vi "LEBITplc.IGSetValue.vi"(0 "i ref in":refnum<vi>, 1 "Nickname in":string, 2 "index in":i32, 3 "value":dbl, 5 "error in (no error)":errorcluster) -> (13 "In Range?":bool, 14 "i ref out":refnum<vi>, 15 "Nicknames out":string[](array[string]), 16 "Index out":i32[](array[numeric]), 17 "values":dbl[](array[numeric]), 18 "Log out":bool[](array[boolean]), 19 "error out":errorcluster)   [LabVIEW 2014, in "LEBITplc.lvlib"]
uses:
  LEBITplc.lvlib
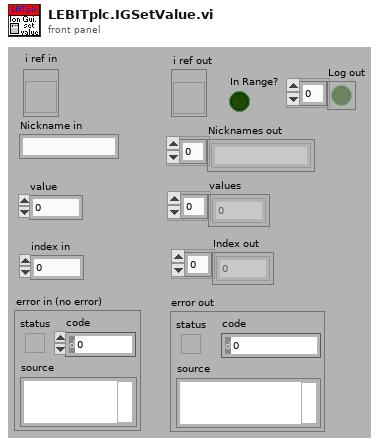
[diagram p1: front panel]
types:
  T1 = typedef "LEBITplc.lvlib/LEBITplc.i attribute.ctl" = cluster{"LLFLocation":string, "SetFileLocation":string, "nickNames":string[], "setValuePLCServiceID":i32[], "GUIServiceID":i32[], "monValuePLC":string[], "SetValueServiceID":i32[], "MonValueServiceID":i32[], "SetValue":dbl[][], "SetValueMin":dbl[], "SetValueMax":dbl[], "SetValueInfoServiceID":i32[], "GUINames":string[], "ListOfBases":string[], "Scale":dbl[], "Offset":dbl[], "setValuePLC":string[], "BaseName":string[], "ScaleServiceID":i32[], "OffsetServiceID":i32[], "AllPLCValues":string[], "CondSpecialArray":string[][], "CondSpecialIndex":i32[], "CondSpecialMonValue":dbl[], "RecentlyChanged":i32[], "SetFileLocationID":i32, "Dependent-Monitors":string[][], "LastLoadedFiles":string[], "IonGuideCalibLocation":string, "Monitor Dependent":string[], "Special":string[], "PLC?":bool[], "Start Date":string, "ListOfBasesServiceID":i32, "SETRA VISA resource":refnum<visa-resource-name>}
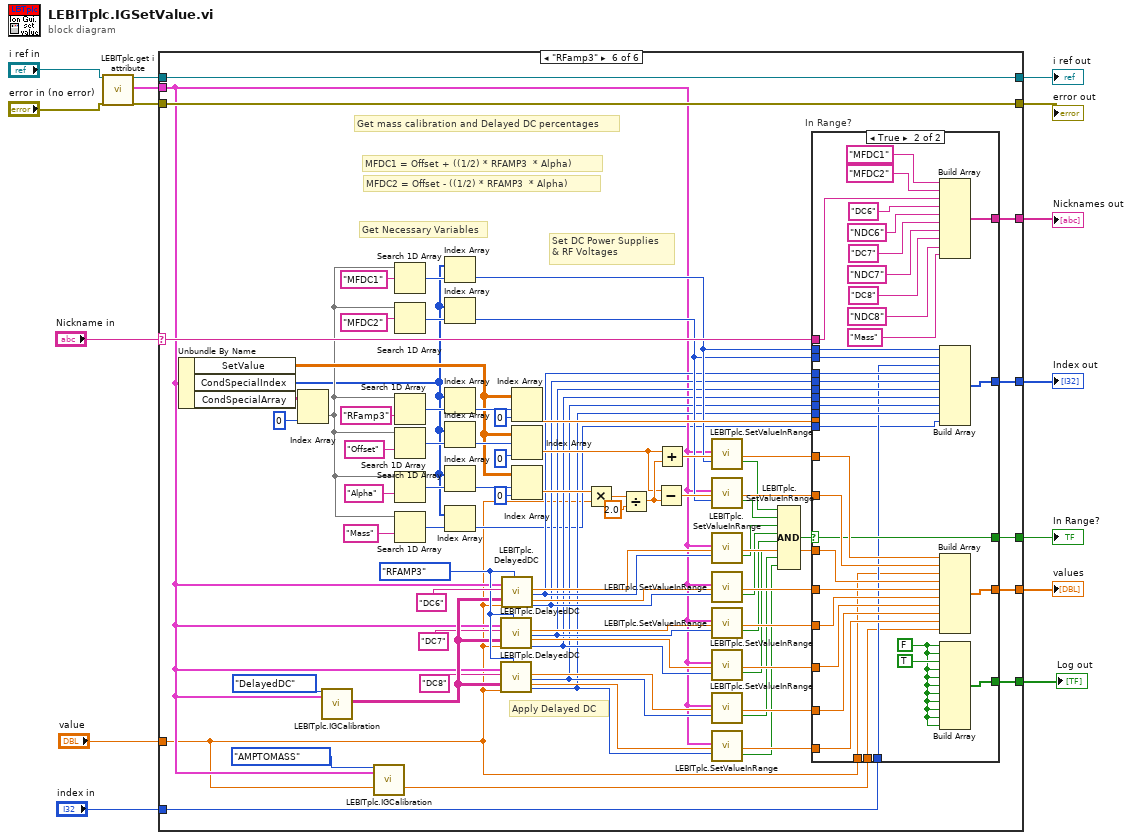
[diagram p0: block diagram]
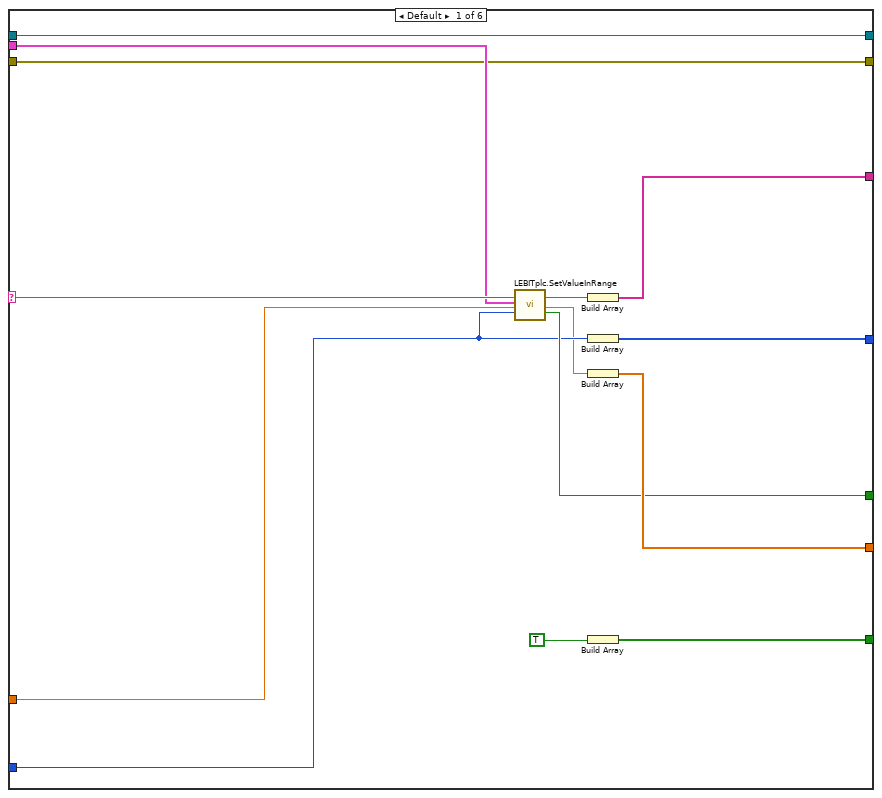
[diagram p2: hidden frame]
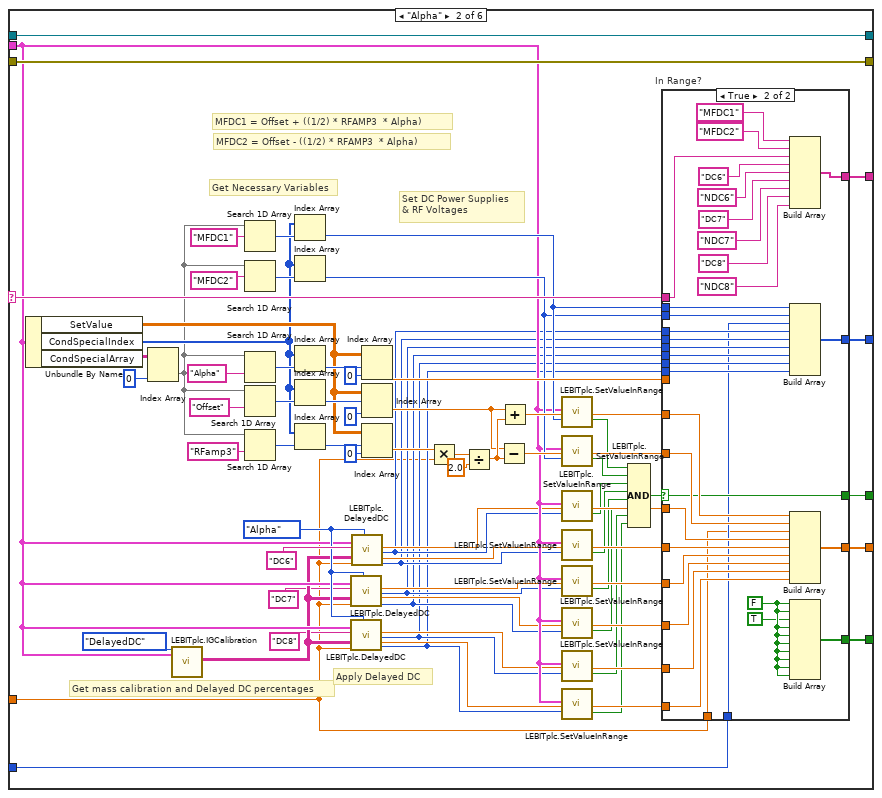
[diagram p3: hidden frame]
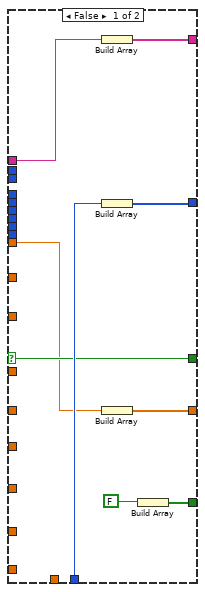
[diagram p4: hidden frame]
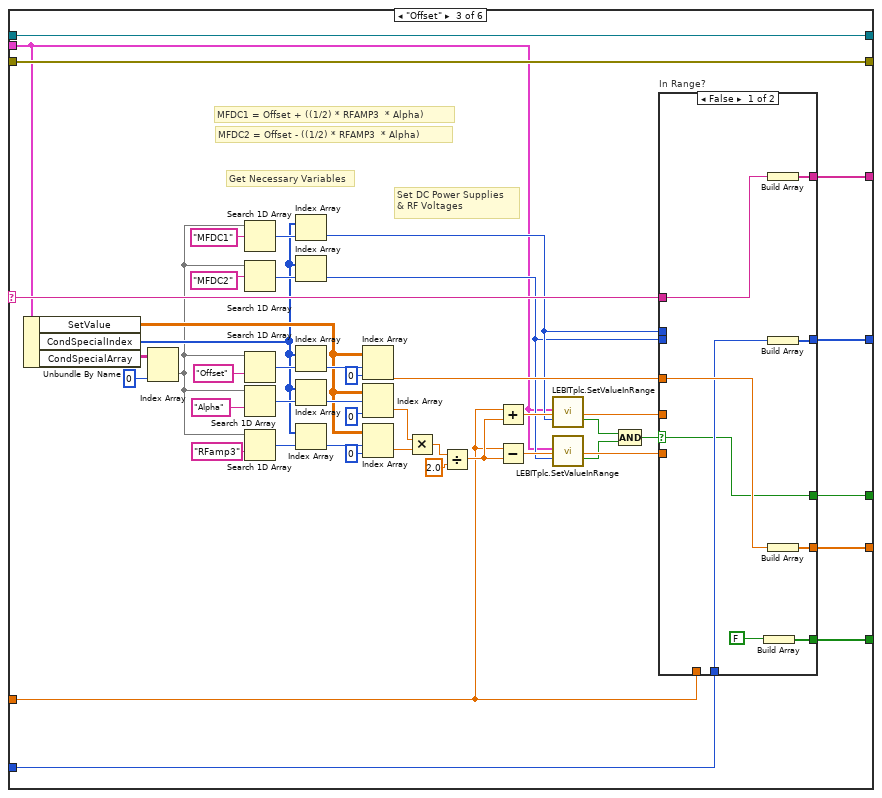
[diagram p5: hidden frame]
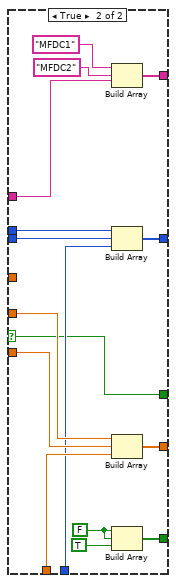
[diagram p6: hidden frame]
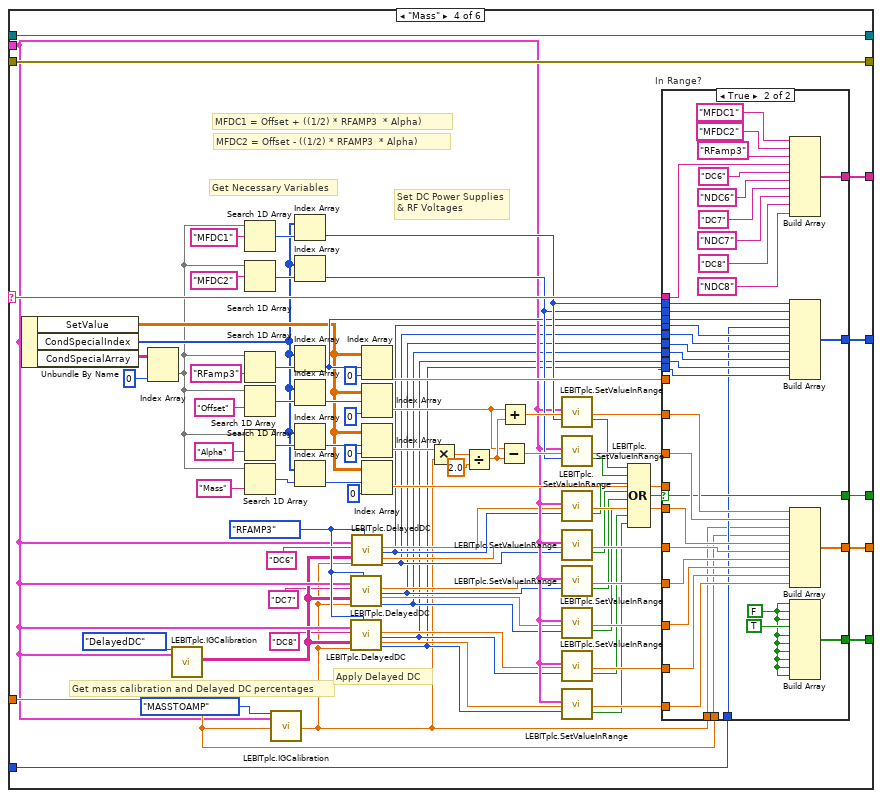
[diagram p7: hidden frame]
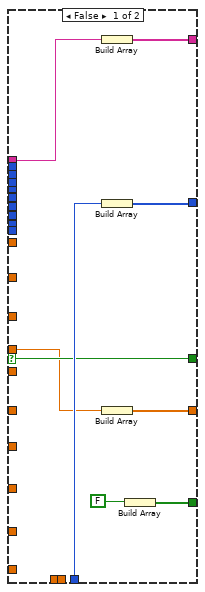
[diagram p8: hidden frame]
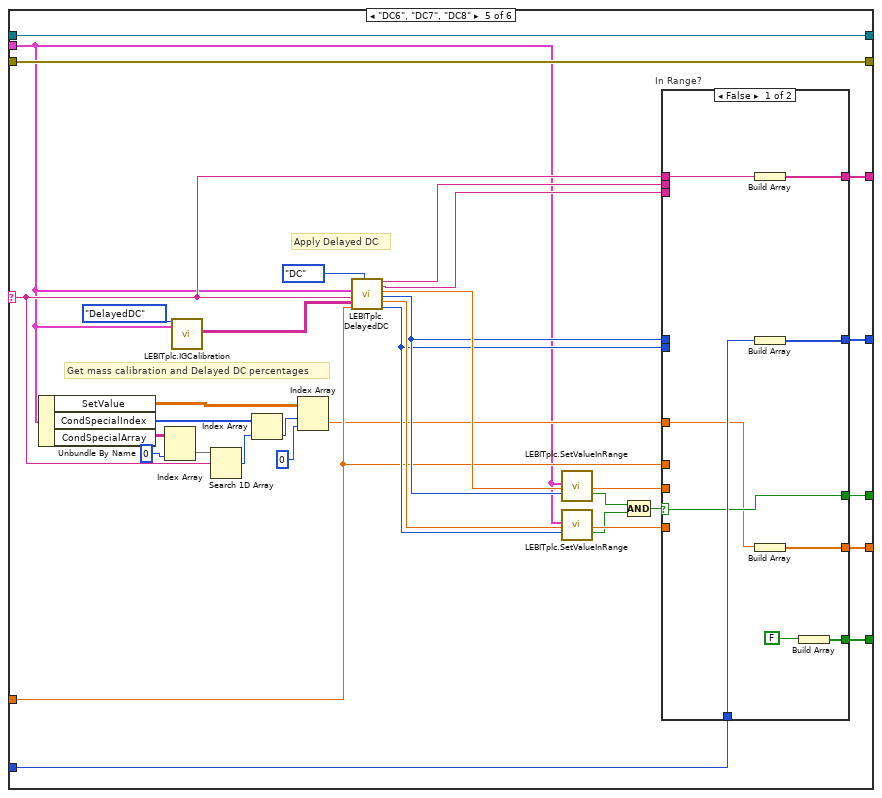
[diagram p9: hidden frame]
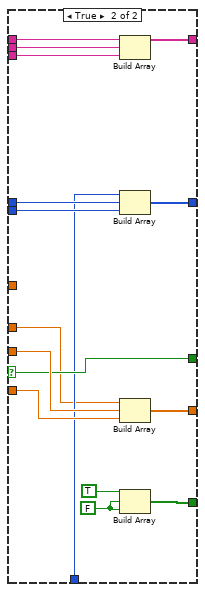
[diagram p10: hidden frame]
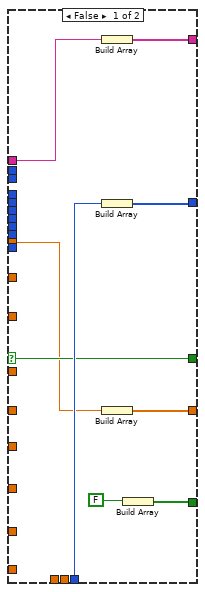
[diagram p11: hidden frame]
diagram:
  n1 = call "LEBITplc.get i attribute.vi"("i ref in"="i ref in", "error in (no error)"="error in (no error)") -> ("i ref out"=w7:refnum<vi>, "i attribute"=w8:T1, "error out"=w6:errorcluster)  [unwired: 15 in]
  n2 = case shown="\"RFamp3\"" "Nickname in" {
    selector: "Nickname in" -> [w25 w92 w182 w291 w353 w478]
    tunnel: w8 -> [w20 w46 w158 w238 w352 w419]
    tunnel: "value" -> [w23 w30 w151 w246 w363 w412]
    tunnel: [w29 w93 w183 w292 w385 w479] -> w13
    tunnel: [w28 w91 w181 w290 w366 w477] -> w12
    tunnel: "index in" -> [w24 w77 w166 w276 w383 w463]
    tunnel: [w27 w80 w169 w279 w384 w466] -> w10
    tunnel: [w26 w75 w164 w274 w382 w461] -> w9
    tunnel: w7 -> [w19 w74 w163 w273 w381 w460]
    tunnel: [w19 w74 w163 w273 w381 w460] -> w3
    tunnel: [w18 w73 w162 w272 w380 w459] -> w2
    tunnel: w6 -> [w18 w73 w162 w272 w380 w459]
    tunnel: [w17 w53 w150 w247 w374 w439] -> w1
    frame Default {
      n3 = call "LEBITplc.SetValueInRange.vi"("CommandName in"=w25, "i attribute in"=w20, "value in"=w23, "index of element"=w24) -> ("CommandName out"=w21:string, "value out"=w22:dbl, "In Range?"=w26:bool)  [unwired: 11 in, 2 out]
      n4 = Build Array(w21) -> (w28:string[])
      n5 = Build Array(w24) -> (w27:i32[])
      n6 = Build Array(w22) -> (w29:dbl[])
      n7 = Build Array(TRUE) -> (w17:bool[])
    }
    frame "Alpha" {
      w47 = enum16{"RFAMP3", "Alpha"}."Alpha" ("Enum")
      # "Get mass calibration and Delayed DC percentages"
      # "Apply Delayed DC"
      # "MFDC2 = Offset - ((1/2) * RFAMP3  * Alpha)"
      # "MFDC1 = Offset + ((1/2) * RFAMP3  * Alpha)"
      # "Set DC Power Supplies \n& RF Voltages"
      # "Get Necessary Variables"
      n8 = Unbundle By Name(w46) -> ("SetValue"=w52:dbl[][], "CondSpecialIndex"=w51:i32[], "CondSpecialArray"=w90:string[][])
      n9 = Index Array(array=w90, index (col)=0 ("index (row)")) -> (element=w50:string[])  [unwired: 1 in]
      n10 = call "LEBITplc.IGCalibration.vi"("Enum"=enum16{"DelayedDC", "MASSTOAMP", "AMPTOMASS"}."DelayedDC", "i attribute"=w46) -> ("Delayed DC"=w45:string[][])  [unwired: 15 in, 2 out]
      n11 = Search 1D Array(1D array=w50, element="MFDC1") -> (index of element=w82:i32)  [unwired: 1 in]
      n12 = Search 1D Array(1D array=w50, element="MFDC2") -> (index of element=w84:i32)  [unwired: 1 in]
      n13 = Search 1D Array(1D array=w50, element="Alpha") -> (index of element=w89:i32)  [unwired: 1 in]
      n14 = Search 1D Array(1D array=w50, element="Offset") -> (index of element=w88:i32)  [unwired: 1 in]
      n15 = Search 1D Array(1D array=w50, element="RFamp3") -> (index of element=w87:i32)  [unwired: 1 in]
      n16 = Index Array(array=w51, index=w82) -> (element=w79:i32)
      n17 = Index Array(array=w51, index=w84) -> (element=w78:i32)
      n18 = Index Array(array=w51, index=w89) -> (element=w54:i32)
      n19 = Index Array(array=w51, index=w88) -> (element=w85:i32)
      n20 = Index Array(array=w51, index=w87) -> (element=w86:i32)
      n21 = call "LEBITplc.DelayedDC.vi"("i attribute"=w46, "Nickname"="DC7", "Delayed DC"=w45, "Value"=w30, "Enum"=w47) -> ("ValuePDC"=w40:dbl, "IndexPDC"=w34:i32, "ValueNDC"=w39:dbl, "IndexNDC"=w33:i32)  [unwired: 9 in, 2 out]
      n22 = call "LEBITplc.DelayedDC.vi"("i attribute"=w46, "Nickname"="DC8", "Delayed DC"=w45, "Value"=w30, "Enum"=w47) -> ("ValuePDC"=w38:dbl, "IndexPDC"=w32:i32, "ValueNDC"=w37:dbl, "IndexNDC"=w31:i32)  [unwired: 9 in, 2 out]
      n23 = call "LEBITplc.DelayedDC.vi"("i attribute"=w46, "Nickname"="DC6", "Delayed DC"=w45, "Value"=w30, "Enum"=w47) -> ("ValuePDC"=w42:dbl, "IndexPDC"=w36:i32, "ValueNDC"=w41:dbl, "IndexNDC"=w35:i32)  [unwired: 9 in, 2 out]
      n24 = Index Array(array=w52, index (row)=w54, index (col)=0 ("disabled index (col)")) -> (element=w98:dbl)
      n25 = Index Array(array=w52, index (row)=w85, index (col)=0 ("disabled index (col)")) -> (element=w55:dbl)
      n26 = Index Array(array=w52, index (row)=w86, index (col)=0 ("disabled index (col)")) -> (element=w56:dbl)
      n27 = Multiply(x=w56, y=w30) -> (x*y=w102:dbl)
      n28 = Divide(x=w102, y=2.0) -> (x/y=w57:dbl)
      n29 = Subtract(x=w55, y=w57) -> (x-y=w97:dbl)
      n30 = Add(x=w55, y=w57) -> (x+y=w96:dbl)
      n31 = call "LEBITplc.SetValueInRange.vi"("i attribute in"=w46, "value in"=w96, "index of element"=w79) -> ("value out"=w94:dbl, "In Range?"=w65:bool)  [unwired: 12 in, 3 out]
      n32 = call "LEBITplc.SetValueInRange.vi"("i attribute in"=w46, "value in"=w97, "index of element"=w78) -> ("value out"=w95:dbl, "In Range?"=w64:bool)  [unwired: 12 in, 3 out]
      n33 = call "LEBITplc.SetValueInRange.vi"("i attribute in"=w46, "value in"=w42, "index of element"=w36) -> ("value out"=w72:dbl, "In Range?"=w63:bool)  [unwired: 12 in, 3 out]
      n34 = call "LEBITplc.SetValueInRange.vi"("i attribute in"=w46, "value in"=w41, "index of element"=w35) -> ("value out"=w71:dbl, "In Range?"=w62:bool)  [unwired: 12 in, 3 out]
      n35 = call "LEBITplc.SetValueInRange.vi"("i attribute in"=w46, "value in"=w40, "index of element"=w34) -> ("value out"=w70:dbl, "In Range?"=w61:bool)  [unwired: 12 in, 3 out]
      n36 = call "LEBITplc.SetValueInRange.vi"("i attribute in"=w46, "value in"=w39, "index of element"=w33) -> ("value out"=w69:dbl, "In Range?"=w60:bool)  [unwired: 12 in, 3 out]
      n37 = call "LEBITplc.SetValueInRange.vi"("i attribute in"=w46, "value in"=w38, "index of element"=w32) -> ("value out"=w68:dbl, "In Range?"=w59:bool)  [unwired: 12 in, 3 out]
      n38 = call "LEBITplc.SetValueInRange.vi"("i attribute in"=w46, "value in"=w37, "index of element"=w31) -> ("value out"=w67:dbl, "In Range?"=w58:bool)  [unwired: 12 in, 3 out]
      n39 = Compound Arithmetic op=AND(w65, w64, w63, w62, w61, w60, w59, w58) -> (w66:bool)
      n40 = case "In Range?" shown="True" w66 {
        selector: w66 -> [w110 w125]
        tunnel: w98 -> [w107 _]
        tunnel: w95 -> [_ w148]
        tunnel: w94 -> [_ w149]
        tunnel: [w115 w147] -> w93
        tunnel: w92 -> [w113 w118]
        tunnel: [w114 w146] -> w91
        tunnel: [w112 w145] -> w80
        tunnel: w79 -> [_ w144]
        tunnel: w78 -> [_ w143]
        tunnel: w77 -> [w111 w121]
        tunnel: [w110 w125] -> w75
        tunnel: w72 -> [_ w131]
        tunnel: w71 -> [_ w129]
        tunnel: w70 -> [_ w130]
        tunnel: w69 -> [_ w128]
        tunnel: w68 -> [_ w127]
        tunnel: w67 -> [_ w126]
        tunnel: w36 -> [_ w122]
        tunnel: w35 -> [_ w142]
        tunnel: w34 -> [_ w141]
        tunnel: w33 -> [_ w140]
        tunnel: w32 -> [_ w139]
        tunnel: w31 -> [_ w138]
        tunnel: w30 -> [_ w120]
        tunnel: [w108 w119] -> w53
        frame False {
          n41 = Build Array(w113) -> (w114:string[])
          n42 = Build Array(w111) -> (w112:i32[])
          n43 = Build Array(w107) -> (w115:dbl[])
          n44 = Build Array(FALSE) -> (w108:bool[])
        }
        frame True {
          w117 = FALSE
          n45 = Build Array("MFDC1" ("element"), "MFDC2" ("element"), w118, "DC6" ("element"), "NDC6" ("element"), "DC7" ("element"), "NDC7" ("element"), "DC8" ("element"), "NDC8" ("element")) -> (w146:string[])
          n46 = Build Array(w144, w143, w121, w122, w142, w141, w140, w139, w138) -> (w145:i32[])
          n47 = Build Array(w149, w148, w120, w131, w129, w130, w128, w127, w126) -> (w147:dbl[])
          n48 = Build Array(w117, w117, TRUE ("element"), w117, w117, w117, w117, w117, w117, w117) -> (w119:bool[])
        }
      }
    }
    frame "Offset" {
      # "MFDC2 = Offset - ((1/2) * RFAMP3  * Alpha)"
      # "MFDC1 = Offset + ((1/2) * RFAMP3  * Alpha)"
      # "Set DC Power Supplies \n& RF Voltages"
      # "Get Necessary Variables"
      n49 = Unbundle By Name(w158) -> ("SetValue"=w161:dbl[][], "CondSpecialIndex"=w160:i32[], "CondSpecialArray"=w180:string[][])
      n50 = Index Array(array=w180, index (col)=0 ("index (row)")) -> (element=w159:string[])  [unwired: 1 in]
      n51 = Search 1D Array(1D array=w159, element="MFDC1") -> (index of element=w171:i32)  [unwired: 1 in]
      n52 = Search 1D Array(1D array=w159, element="MFDC2") -> (index of element=w173:i32)  [unwired: 1 in]
      n53 = Search 1D Array(1D array=w159, element="Offset") -> (index of element=w179:i32)  [unwired: 1 in]
      n54 = Search 1D Array(1D array=w159, element="Alpha") -> (index of element=w178:i32)  [unwired: 1 in]
      n55 = Search 1D Array(1D array=w159, element="RFamp3") -> (index of element=w177:i32)  [unwired: 1 in]
      n56 = Index Array(array=w160, index=w171) -> (element=w168:i32)
      n57 = Index Array(array=w160, index=w173) -> (element=w167:i32)
      n58 = Index Array(array=w160, index=w179) -> (element=w174:i32)
      n59 = Index Array(array=w160, index=w178) -> (element=w175:i32)
      n60 = Index Array(array=w160, index=w177) -> (element=w176:i32)
      n61 = Index Array(array=w161, index (row)=w174, index (col)=0 ("disabled index (col)")) -> (element=w188:dbl)
      n62 = Index Array(array=w161, index (row)=w175, index (col)=0 ("disabled index (col)")) -> (element=w154:dbl)
      n63 = Index Array(array=w161, index (row)=w176, index (col)=0 ("disabled index (col)")) -> (element=w153:dbl)
      n64 = Multiply(x=w154, y=w153) -> (x*y=w192:dbl)
      n65 = Divide(x=w192, y=2.0) -> (x/y=w152:dbl)
      n66 = Add(x=w151, y=w152) -> (x+y=w186:dbl)
      n67 = Subtract(x=w151, y=w152) -> (x-y=w187:dbl)
      n68 = call "LEBITplc.SetValueInRange.vi"("i attribute in"=w158, "value in"=w186, "index of element"=w168) -> ("value out"=w184:dbl, "In Range?"=w156:bool)  [unwired: 12 in, 3 out]
      n69 = call "LEBITplc.SetValueInRange.vi"("i attribute in"=w158, "value in"=w187, "index of element"=w167) -> ("value out"=w185:dbl, "In Range?"=w155:bool)  [unwired: 12 in, 3 out]
      n70 = Compound Arithmetic op=AND(w156, w155) -> (w157:bool)
      n71 = case "In Range?" shown="False" w157 {
        selector: w157 -> [w199 w209]
        tunnel: w188 -> [w205 _]
        tunnel: w151 -> [_ w219]
        tunnel: w185 -> [_ w220]
        tunnel: w184 -> [_ w221]
        tunnel: [w204 w218] -> w183
        tunnel: w182 -> [w202 w210]
        tunnel: [w203 w215] -> w181
        tunnel: [w201 w214] -> w169
        tunnel: w168 -> [_ w213]
        tunnel: w167 -> [_ w212]
        tunnel: w166 -> [w200 w211]
        tunnel: [w199 w209] -> w164
        tunnel: [w197 w208] -> w150
        frame False {
          n72 = Build Array(FALSE) -> (w197:bool[])
          n73 = Build Array(w202) -> (w203:string[])
          n74 = Build Array(w200) -> (w201:i32[])
          n75 = Build Array(w205) -> (w204:dbl[])
        }
        frame True {
          w206 = FALSE
          n76 = Build Array("MFDC1" ("element"), "MFDC2" ("element"), w210) -> (w215:string[])
          n77 = Build Array(w213, w212, w211) -> (w214:i32[])
          n78 = Build Array(w221, w220, w219) -> (w218:dbl[])
          n79 = Build Array(w206, w206, TRUE ("element")) -> (w208:bool[])
        }
      }
    }
    frame "Mass" {
      w239 = enum16{"RFAMP3", "Alpha"}."RFAMP3" ("Enum")
      # "Get mass calibration and Delayed DC percentages"
      # "Apply Delayed DC"
      # "MFDC2 = Offset - ((1/2) * RFAMP3  * Alpha)"
      # "MFDC1 = Offset + ((1/2) * RFAMP3  * Alpha)"
      # "Set DC Power Supplies \n& RF Voltages"
      # "Get Necessary Variables"
      n80 = Unbundle By Name(w238) -> ("SetValue"=w245:dbl[][], "CondSpecialIndex"=w244:i32[], "CondSpecialArray"=w289:string[][])
      n81 = Index Array(array=w289, index (col)=0 ("index (row)")) -> (element=w243:string[])  [unwired: 1 in]
      n82 = call "LEBITplc.IGCalibration.vi"("Enum"=enum16{"DelayedDC", "MASSTOAMP", "AMPTOMASS"}."DelayedDC", "i attribute"=w238) -> ("Delayed DC"=w237:string[][])  [unwired: 15 in, 2 out]
      n83 = Search 1D Array(1D array=w243, element="MFDC1") -> (index of element=w281:i32)  [unwired: 1 in]
      n84 = Search 1D Array(1D array=w243, element="MFDC2") -> (index of element=w283:i32)  [unwired: 1 in]
      n85 = Search 1D Array(1D array=w243, element="RFamp3") -> (index of element=w288:i32)  [unwired: 1 in]
      n86 = Search 1D Array(1D array=w243, element="Offset") -> (index of element=w287:i32)  [unwired: 1 in]
      n87 = Search 1D Array(1D array=w243, element="Alpha") -> (index of element=w286:i32)  [unwired: 1 in]
      n88 = Search 1D Array(1D array=w243, element="Mass") -> (index of element=w252:i32)  [unwired: 1 in]
      n89 = call "LEBITplc.IGCalibration.vi"("Enum"=enum16{"DelayedDC", "MASSTOAMP", "AMPTOMASS"}."MASSTOAMP", "i attribute"=w238, "MASS"=w246) -> ("AMP"=w222:dbl)  [unwired: 14 in, 2 out]
      n90 = Index Array(array=w244, index=w281) -> (element=w278:i32)
      n91 = Index Array(array=w244, index=w283) -> (element=w277:i32)
      n92 = Index Array(array=w244, index=w288) -> (element=w249:i32)
      n93 = Index Array(array=w244, index=w287) -> (element=w284:i32)
      n94 = Index Array(array=w244, index=w286) -> (element=w285:i32)
      n95 = Index Array(array=w244, index=w252) -> (element=w250:i32)
      n96 = call "LEBITplc.DelayedDC.vi"("i attribute"=w238, "Nickname"="DC7", "Delayed DC"=w237, "Value"=w222, "Enum"=w239) -> ("ValuePDC"=w232:dbl, "IndexPDC"=w226:i32, "ValueNDC"=w231:dbl, "IndexNDC"=w225:i32)  [unwired: 9 in, 2 out]
      n97 = call "LEBITplc.DelayedDC.vi"("i attribute"=w238, "Nickname"="DC8", "Delayed DC"=w237, "Value"=w222, "Enum"=w239) -> ("ValuePDC"=w230:dbl, "IndexPDC"=w224:i32, "ValueNDC"=w229:dbl, "IndexNDC"=w223:i32)  [unwired: 9 in, 2 out]
      n98 = call "LEBITplc.DelayedDC.vi"("i attribute"=w238, "Nickname"="DC6", "Delayed DC"=w237, "Value"=w222, "Enum"=w239) -> ("ValuePDC"=w234:dbl, "IndexPDC"=w228:i32, "ValueNDC"=w233:dbl, "IndexNDC"=w227:i32)  [unwired: 9 in, 2 out]
      n99 = Index Array(array=w245, index (row)=w249, index (col)=0 ("disabled index (col)")) -> (element=w297:dbl)
      n100 = Index Array(array=w245, index (row)=w284, index (col)=0 ("disabled index (col)")) -> (element=w254:dbl)
      n101 = Index Array(array=w245, index (row)=w285, index (col)=0 ("disabled index (col)")) -> (element=w255:dbl)
      n102 = Index Array(array=w245, index (row)=w250, index (col)=0 ("disabled index (col)")) -> (element=w248:dbl)
      n103 = Multiply(x=w255, y=w222) -> (x*y=w301:dbl)
      n104 = Divide(x=w301, y=2.0) -> (x/y=w256:dbl)
      n105 = Subtract(x=w254, y=w256) -> (x-y=w296:dbl)
      n106 = Add(x=w254, y=w256) -> (x+y=w295:dbl)
      n107 = call "LEBITplc.SetValueInRange.vi"("i attribute in"=w238, "value in"=w295, "index of element"=w278) -> ("value out"=w293:dbl, "In Range?"=w264:bool)  [unwired: 12 in, 3 out]
      n108 = call "LEBITplc.SetValueInRange.vi"("i attribute in"=w238, "value in"=w296, "index of element"=w277) -> ("value out"=w294:dbl, "In Range?"=w263:bool)  [unwired: 12 in, 3 out]
      n109 = call "LEBITplc.SetValueInRange.vi"("i attribute in"=w238, "value in"=w234, "index of element"=w228) -> ("value out"=w271:dbl, "In Range?"=w262:bool)  [unwired: 12 in, 3 out]
      n110 = call "LEBITplc.SetValueInRange.vi"("i attribute in"=w238, "value in"=w233, "index of element"=w227) -> ("value out"=w270:dbl, "In Range?"=w261:bool)  [unwired: 12 in, 3 out]
      n111 = call "LEBITplc.SetValueInRange.vi"("i attribute in"=w238, "value in"=w232, "index of element"=w226) -> ("value out"=w269:dbl, "In Range?"=w260:bool)  [unwired: 12 in, 3 out]
      n112 = call "LEBITplc.SetValueInRange.vi"("i attribute in"=w238, "value in"=w231, "index of element"=w225) -> ("value out"=w268:dbl, "In Range?"=w259:bool)  [unwired: 12 in, 3 out]
      n113 = call "LEBITplc.SetValueInRange.vi"("i attribute in"=w238, "value in"=w230, "index of element"=w224) -> ("value out"=w267:dbl, "In Range?"=w258:bool)  [unwired: 12 in, 3 out]
      n114 = call "LEBITplc.SetValueInRange.vi"("i attribute in"=w238, "value in"=w229, "index of element"=w223) -> ("value out"=w266:dbl, "In Range?"=w257:bool)  [unwired: 12 in, 3 out]
      n115 = Compound Arithmetic op=OR(w264, w263, w262, w261, w260, w259, w258, w257) -> (w265:bool)
      n116 = case "In Range?" shown="True" w265 {
        selector: w265 -> [w309 w327]
        tunnel: w297 -> [_ _]
        tunnel: w248 -> [w308 _]
        tunnel: w294 -> [_ w350]
        tunnel: w293 -> [_ w351]
        tunnel: [w314 w349] -> w292
        tunnel: w291 -> [w312 w323]
        tunnel: [w313 w348] -> w290
        tunnel: [w311 w347] -> w279
        tunnel: w278 -> [_ w346]
        tunnel: w277 -> [_ w345]
        tunnel: w276 -> [w310 w321]
        tunnel: [w309 w327] -> w274
        tunnel: w271 -> [_ w333]
        tunnel: w270 -> [_ w331]
        tunnel: w269 -> [_ w332]
        tunnel: w268 -> [_ w330]
        tunnel: w267 -> [_ w329]
        tunnel: w266 -> [_ w328]
        tunnel: w228 -> [_ w322]
        tunnel: w227 -> [_ w344]
        tunnel: w226 -> [_ w343]
        tunnel: w225 -> [_ w342]
        tunnel: w224 -> [_ w341]
        tunnel: w223 -> [_ w340]
        tunnel: w249 -> [_ w320]
        tunnel: w222 -> [_ w319]
        tunnel: w246 -> [_ w318]
        tunnel: [w306 w315] -> w247
        frame False {
          n117 = Build Array(w312) -> (w313:string[])
          n118 = Build Array(w310) -> (w311:i32[])
          n119 = Build Array(w308) -> (w314:dbl[])
          n120 = Build Array(FALSE) -> (w306:bool[])
        }
        frame True {
          w316 = FALSE
          n121 = Build Array("MFDC1" ("element"), "MFDC2" ("element"), "RFamp3" ("element"), w323, "DC6" ("element"), "NDC6" ("element"), "DC7" ("element"), "NDC7" ("element"), "DC8" ("element"), "NDC8" ("element")) -> (w348:string[])
          n122 = Build Array(w346, w345, w320, w321, w322, w344, w343, w342, w341, w340) -> (w347:i32[])
          n123 = Build Array(w351, w350, w319, w318, w333, w331, w332, w330, w329, w328) -> (w349:dbl[])
          n124 = Build Array(w316, w316, w316, TRUE ("element"), w316, w316, w316, w316, w316, w316) -> (w315:bool[])
        }
      }
    }
    frame "DC6", "DC7", "DC8" {
      # "Get mass calibration and Delayed DC percentages"
      # "Apply Delayed DC"
      n125 = Unbundle By Name(w352) -> ("SetValue"=w357:dbl[][], "CondSpecialIndex"=w359:i32[], "CondSpecialArray"=w362:string[][])
      n126 = Index Array(array=w362, index (col)=0 ("index (row)")) -> (element=w360:string[])  [unwired: 1 in]
      n127 = call "LEBITplc.IGCalibration.vi"("Enum"=enum16{"DelayedDC", "MASSTOAMP", "AMPTOMASS"}."DelayedDC", "i attribute"=w352) -> ("Delayed DC"=w372:string[][])  [unwired: 15 in, 2 out]
      n128 = Search 1D Array(1D array=w360, element=w353) -> (index of element=w358:i32)  [unwired: 1 in]
      n129 = Index Array(array=w359, index=w358) -> (element=w356:i32)
      n130 = Index Array(array=w357, index (row)=w356, index (col)=0 ("disabled index (col)")) -> (element=w354:dbl)
      n131 = call "LEBITplc.DelayedDC.vi"("i attribute"=w352, "Nickname"=w353, "Delayed DC"=w372, "Value"=w363, "Enum"=enum16{"RFAMP3", "Alpha", "DC"}."DC") -> ("NicknamePDC"=w365:string, "NicknameNDC"=w364:string, "ValuePDC"=w371:dbl, "IndexPDC"=w369:i32, "ValueNDC"=w370:dbl, "IndexNDC"=w368:i32)  [unwired: 9 in]
      n132 = call "LEBITplc.SetValueInRange.vi"("i attribute in"=w352, "value in"=w371, "index of element"=w369) -> ("value out"=w379:dbl, "In Range?"=w376:bool)  [unwired: 12 in, 3 out]
      n133 = call "LEBITplc.SetValueInRange.vi"("i attribute in"=w352, "value in"=w370, "index of element"=w368) -> ("value out"=w378:dbl, "In Range?"=w375:bool)  [unwired: 12 in, 3 out]
      n134 = Compound Arithmetic op=AND(w376, w375) -> (w377:bool)
      n135 = case "In Range?" shown="False" w377 {
        selector: w377 -> [w392 w404]
        tunnel: [w389 w410] -> w385
        tunnel: [w391 w409] -> w366
        tunnel: [w394 w408] -> w384
        tunnel: w383 -> [w393 w402]
        tunnel: [w392 w404] -> w382
        tunnel: w379 -> [_ w406]
        tunnel: w378 -> [_ w405]
        tunnel: w369 -> [_ w403]
        tunnel: w368 -> [_ w407]
        tunnel: w363 -> [_ w401]
        tunnel: [w386 w399] -> w374
        tunnel: w353 -> [w390 w398]
        tunnel: w365 -> [_ w397]
        tunnel: w364 -> [_ w396]
        tunnel: w354 -> [w388 _]
        frame False {
          n136 = Build Array(w390) -> (w391:string[])
          n137 = Build Array(w393) -> (w394:i32[])
          n138 = Build Array(w388) -> (w389:dbl[])
          n139 = Build Array(FALSE) -> (w386:bool[])
        }
        frame True {
          w400 = FALSE
          n140 = Build Array(w398, w397, w396) -> (w409:string[])
          n141 = Build Array(w402, w403, w407) -> (w408:i32[])
          n142 = Build Array(w401, w406, w405) -> (w410:dbl[])
          n143 = Build Array(TRUE ("element"), w400, w400) -> (w399:bool[])
        }
      }
    }
    frame "RFamp3" {
      w435 = enum16{"RFAMP3", "Alpha"}."RFAMP3" ("Enum")
      # "Get mass calibration and Delayed DC percentages"
      # "Apply Delayed DC"
      # "MFDC2 = Offset - ((1/2) * RFAMP3  * Alpha)"
      # "MFDC1 = Offset + ((1/2) * RFAMP3  * Alpha)"
      # "Set DC Power Supplies \n& RF Voltages"
      # "Get Necessary Variables"
      n144 = Unbundle By Name(w419) -> ("SetValue"=w438:dbl[][], "CondSpecialIndex"=w414:i32[], "CondSpecialArray"=w476:string[][])
      n145 = Index Array(array=w476, index (col)=0 ("index (row)")) -> (element=w415:string[])  [unwired: 1 in]
      n146 = call "LEBITplc.IGCalibration.vi"("Enum"=enum16{"DelayedDC", "MASSTOAMP", "AMPTOMASS"}."DelayedDC", "i attribute"=w419) -> ("Delayed DC"=w434:string[][])  [unwired: 15 in, 2 out]
      n147 = call "LEBITplc.IGCalibration.vi"("Enum"=enum16{"DelayedDC", "MASSTOAMP", "AMPTOMASS"}."AMPTOMASS", "i attribute"=w419, "AMP"=w412) -> ("MASS"=w411:dbl)  [unwired: 14 in, 2 out]
      n148 = Search 1D Array(1D array=w415, element="MFDC1") -> (index of element=w468:i32)  [unwired: 1 in]
      n149 = Search 1D Array(1D array=w415, element="MFDC2") -> (index of element=w470:i32)  [unwired: 1 in]
      n150 = Search 1D Array(1D array=w415, element="RFamp3") -> (index of element=w475:i32)  [unwired: 1 in]
      n151 = Search 1D Array(1D array=w415, element="Offset") -> (index of element=w474:i32)  [unwired: 1 in]
      n152 = Search 1D Array(1D array=w415, element="Alpha") -> (index of element=w473:i32)  [unwired: 1 in]
      n153 = Search 1D Array(1D array=w415, element="Mass") -> (index of element=w416:i32)  [unwired: 1 in]
      n154 = Index Array(array=w414, index=w468) -> (element=w465:i32)
      n155 = Index Array(array=w414, index=w470) -> (element=w464:i32)
      n156 = Index Array(array=w414, index=w475) -> (element=w440:i32)
      n157 = Index Array(array=w414, index=w474) -> (element=w471:i32)
      n158 = Index Array(array=w414, index=w473) -> (element=w472:i32)
      n159 = Index Array(array=w414, index=w416) -> (element=w413:i32)
      n160 = call "LEBITplc.DelayedDC.vi"("i attribute"=w419, "Nickname"="DC7", "Delayed DC"=w434, "Value"=w412, "Enum"=w435) -> ("ValuePDC"=w429:dbl, "IndexPDC"=w423:i32, "ValueNDC"=w428:dbl, "IndexNDC"=w422:i32)  [unwired: 9 in, 2 out]
      n161 = call "LEBITplc.DelayedDC.vi"("i attribute"=w419, "Nickname"="DC8", "Delayed DC"=w434, "Value"=w412, "Enum"=w435) -> ("ValuePDC"=w427:dbl, "IndexPDC"=w421:i32, "ValueNDC"=w426:dbl, "IndexNDC"=w420:i32)  [unwired: 9 in, 2 out]
      n162 = call "LEBITplc.DelayedDC.vi"("i attribute"=w419, "Nickname"="DC6", "Delayed DC"=w434, "Value"=w412, "Enum"=w435) -> ("ValuePDC"=w431:dbl, "IndexPDC"=w425:i32, "ValueNDC"=w430:dbl, "IndexNDC"=w424:i32)  [unwired: 9 in, 2 out]
      n163 = Index Array(array=w438, index (row)=w440, index (col)=0 ("disabled index (col)")) -> (element=w484:dbl)
      n164 = Index Array(array=w438, index (row)=w471, index (col)=0 ("disabled index (col)")) -> (element=w441:dbl)
      n165 = Index Array(array=w438, index (row)=w472, index (col)=0 ("disabled index (col)")) -> (element=w442:dbl)
      n166 = Multiply(x=w442, y=w412) -> (x*y=w488:dbl)
      n167 = Divide(x=w488, y=2.0) -> (x/y=w443:dbl)
      n168 = Subtract(x=w441, y=w443) -> (x-y=w483:dbl)
      n169 = Add(x=w441, y=w443) -> (x+y=w482:dbl)
      n170 = call "LEBITplc.SetValueInRange.vi"("i attribute in"=w419, "value in"=w482, "index of element"=w465) -> ("value out"=w480:dbl, "In Range?"=w451:bool)  [unwired: 12 in, 3 out]
      n171 = call "LEBITplc.SetValueInRange.vi"("i attribute in"=w419, "value in"=w483, "index of element"=w464) -> ("value out"=w481:dbl, "In Range?"=w450:bool)  [unwired: 12 in, 3 out]
      n172 = call "LEBITplc.SetValueInRange.vi"("i attribute in"=w419, "value in"=w431, "index of element"=w425) -> ("value out"=w458:dbl, "In Range?"=w449:bool)  [unwired: 12 in, 3 out]
      n173 = call "LEBITplc.SetValueInRange.vi"("i attribute in"=w419, "value in"=w430, "index of element"=w424) -> ("value out"=w457:dbl, "In Range?"=w448:bool)  [unwired: 12 in, 3 out]
      n174 = call "LEBITplc.SetValueInRange.vi"("i attribute in"=w419, "value in"=w429, "index of element"=w423) -> ("value out"=w456:dbl, "In Range?"=w447:bool)  [unwired: 12 in, 3 out]
      n175 = call "LEBITplc.SetValueInRange.vi"("i attribute in"=w419, "value in"=w428, "index of element"=w422) -> ("value out"=w455:dbl, "In Range?"=w446:bool)  [unwired: 12 in, 3 out]
      n176 = call "LEBITplc.SetValueInRange.vi"("i attribute in"=w419, "value in"=w427, "index of element"=w421) -> ("value out"=w454:dbl, "In Range?"=w445:bool)  [unwired: 12 in, 3 out]
      n177 = call "LEBITplc.SetValueInRange.vi"("i attribute in"=w419, "value in"=w426, "index of element"=w420) -> ("value out"=w453:dbl, "In Range?"=w444:bool)  [unwired: 12 in, 3 out]
      n178 = Compound Arithmetic op=AND(w451, w450, w449, w448, w447, w446, w445, w444) -> (w452:bool)
      n179 = case "In Range?" shown="True" w452 {
        selector: w452 -> [w496 w514]
        tunnel: w484 -> [w493 _]
        tunnel: w481 -> [_ w537]
        tunnel: w480 -> [_ w538]
        tunnel: [w501 w536] -> w479
        tunnel: w478 -> [w499 w507]
        tunnel: [w500 w535] -> w477
        tunnel: [w498 w534] -> w466
        tunnel: w465 -> [_ w533]
        tunnel: w464 -> [_ w532]
        tunnel: w463 -> [w497 w510]
        tunnel: [w496 w514] -> w461
        tunnel: w458 -> [_ w520]
        tunnel: w457 -> [_ w518]
        tunnel: w456 -> [_ w519]
        tunnel: w455 -> [_ w517]
        tunnel: w454 -> [_ w516]
        tunnel: w453 -> [_ w515]
        tunnel: w425 -> [_ w511]
        tunnel: w424 -> [_ w531]
        tunnel: w423 -> [_ w530]
        tunnel: w422 -> [_ w529]
        tunnel: w421 -> [_ w528]
        tunnel: w420 -> [_ w527]
        tunnel: w412 -> [_ w509]
        tunnel: [w495 w508] -> w439
        tunnel: w413 -> [_ w504]
        tunnel: w411 -> [_ w503]
        frame False {
          n180 = Build Array(w499) -> (w500:string[])
          n181 = Build Array(w497) -> (w498:i32[])
          n182 = Build Array(w493) -> (w501:dbl[])
          n183 = Build Array(FALSE) -> (w495:bool[])
        }
        frame True {
          w502 = FALSE
          n184 = Build Array("MFDC1" ("element"), "MFDC2" ("element"), w507, "DC6" ("element"), "NDC6" ("element"), "DC7" ("element"), "NDC7" ("element"), "DC8" ("element"), "NDC8" ("element"), "Mass" ("element")) -> (w535:string[])
          n185 = Build Array(w533, w532, w510, w511, w531, w530, w529, w528, w527, w504) -> (w534:i32[])
          n186 = Build Array(w538, w537, w509, w520, w518, w519, w517, w516, w515, w503) -> (w536:dbl[])
          n187 = Build Array(w502, w502, TRUE ("element"), w502, w502, w502, w502, w502, w502, w502, w502) -> (w508:bool[])
        }
      }
    }
  }
  "values" <- w13
  "Nicknames out" <- w12
  "Index out" <- w10
  "In Range?" <- w9
  "i ref out" <- w3
  "error out" <- w2
  "Log out" <- w1
